vi "ScaleParamData.vi"(1 "max scale value":i16, 2 "parameter":u16(ring) items=["midband", "slope", "intercept"], 3 "Range Params":T1={"mb max"=-10.0, "mb min"=-60.0, "slope max"=4.0, "slope min"=-8.0, "int max"=5.0, "int min"=-85.0} {"int min" format="%.2f"; "int max" format="%.2f"; "slope min" format="%.2f"; "slope max" format="%.2f"; "mb min" format="%.2f"; "mb max" format="%.2f"}, 4 "raw image data in":dbl[][](array[numeric]) format="%.2f") -> (0 "scaled output":dbl[][](array[numeric]))   [LabVIEW 2022 SP3]
uses:
  <vilib>/Analysis/NI_AALPro.lvlib
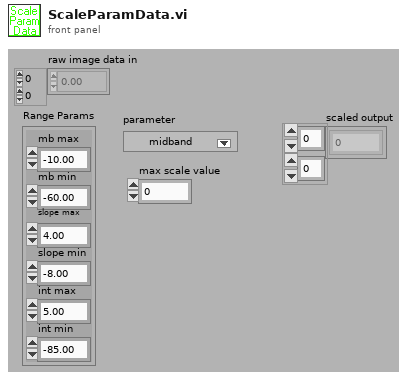
[diagram p1: front panel]
types:
  T1 = cluster{"mb max":dbl, "mb min":dbl, "slope max":dbl, "slope min":dbl, "int max":dbl, "int min":dbl}
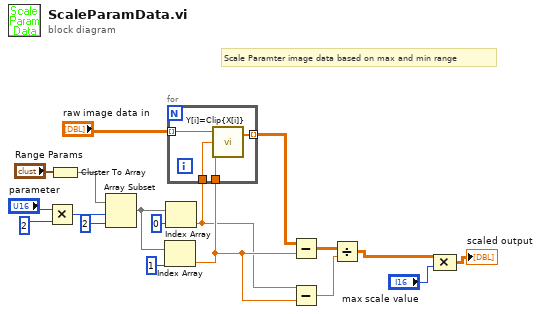
[diagram p0: block diagram]
diagram:
  # "Scale Paramter image data based on max and min range"
  n1 = Multiply(x="parameter", y=2) -> (x*y=w15:i32)
  n2 = Cluster To Array(cluster="Range Params") -> (array=w16:dbl[])
  n3 = Array Subset(array=w16, index=w15, length=2) -> (w12:dbl[])
  n4 = Index Array(array=w12, index=1) -> (element=w5:dbl)
  n5 = Index Array(array=w12, index=0) -> (element=w3:dbl)
  n6 = for {
    tunnel: "raw image data in" -> [w22] mode=indexing
    tunnel: w5 -> [w21]
    tunnel: w3 -> [w20]
    tunnel: [w19] -> w4 mode=indexing
    n7 = call <vilib>:"Y[i]=Clip{X[i]}.vi"("lower limit"=w21, "upper limit"=w20, "Input Array"=w22) -> ("Clipped Array"=w19:dbl[])  [unwired: 1 out]
  }
  n8 = Subtract(x=w4, y=w5) -> (x-y=w7:dbl[][])
  n9 = Subtract(x=w3, y=w5) -> (x-y=w6:dbl)
  n10 = Divide(x=w7, y=w6) -> (x/y=w1:dbl[][])
  n11 = Compound Arithmetic op=MULTIPLY(w1, "max scale value") -> (→"scaled output":dbl[][])
